vi "Stream Wait for Input.vi"   [LabVIEW 2013, in "Zaber A Series.lvlib"]
doc: "Causes stream processing to pause until an analog or digital input condition has been met. The controller will monitor its input pins until the condition is satisfied.\n\nIf the Reference Value input is connected to a boolean, digital inputs will be monitored. If the reference value is numeric, analog inputs will be monitored.\n\nThis VI does not check in advance for error conditions such as streams not being supported.\n\nThis VI requires that the Initialize VI has been called with the same serial port and that the specified stream buffer has already been opened."
uses:
  Zaber A Series.lvlib
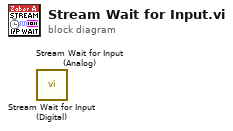
[diagram p0: block diagram]
diagram:
  n1 = call "Stream Wait for Input (Digital).vi"() -> ()  [unwired: 10 in, 2 out]
  n2 = call "Stream Wait for Input (Analog).vi"() -> ()  [unwired: 10 in, 2 out]
